vi "Directional Speed Sensor Page - Multi FPGA.vi"(8 "error in (no error)":errorcluster, 11 "Node Ptr":T1 format="%.0x") -> (0 "error out":errorcluster)   [LabVIEW 2015, in "Engine Simulation Toolkit System Explorer.lvlib"]
uses:
  <vilib>/NI Veristand/Custom Device API/Custom Device Item Ref.ctl
  Shared/Properties.vi
  Shared/Constants and GUIDs.vi
  <vilib>/NI Veristand/Custom Device Tools/Custom Device Utility Library/NI VeriStand - Search for All Items by GUID.vi
  <vilib>/NI Veristand/Custom Device API/Set Item Property (Dependent Node Pointer).vi
  <vilib>/NI Veristand/Custom Device API/Get Item Property (String).vi
  <vilib>/NI Veristand/Custom Device API/Get Item Property (Dependent Node Pointer).vi
  Engine Simulation Toolkit System Explorer.lvlib
  <vilib>/NI Veristand/Custom Device API/Custom Device API.lvlib
  Shared/Engine Simulation Toolkit Shared.lvlib
  <vilib>/NI Veristand/Custom Device Tools/Custom Device Utility Library/Custom Device Utility Library.lvlib
panel:
  in  "ToothSource":u16(ring) caption="Digital pattern to use for tooth centers"
  in  "Tr (uS)":dbl min=0.0 max=1638.4 step=0.025
  in  "Tf (uS)":dbl min=0.0 max=1638.4 step=0.025
  in  "Td (uS)":dbl min=0.0 max=1638.4 step=0.025
  out "Name in bitfile":string
  in  "Name":string
  in  "Header":cluster{"Section Name":string}={"Section Name"="Directional Speed Sensor Settings"}
  # "(Delay time)"
  # "(Forward pulse duration)"
  # "(Reverse pulse duration)"
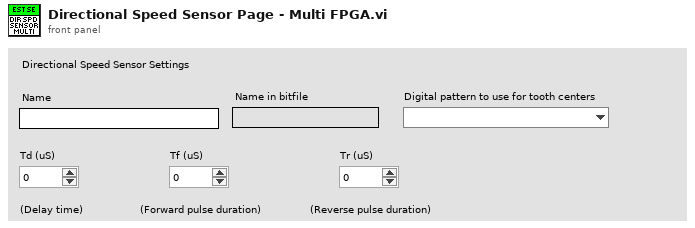
[diagram p1: front panel]
types:
  T1 = typedef "Custom Device API.lvlib/Custom Device Item Ref.ctl" = u64
  T2 = typedef "Engine Simulation Toolkit Shared.lvlib/Channel.ctl" = cluster{"Name":string, "Units":string, "Default":dbl, "Description":string, "Scalable":bool}
  T3 = typedef "Custom Device API.lvlib/Custom Device Item Info.ctl" = cluster{"Name":string, "Is Channel":bool, "GUID":string, "Is Waveform":bool}
  T4 = typedef "Custom Device API.lvlib/Custom Device Commands.ctl" = enum16{"Default", "Item renamed", "Shutdown", "Dynamic button pressed"}
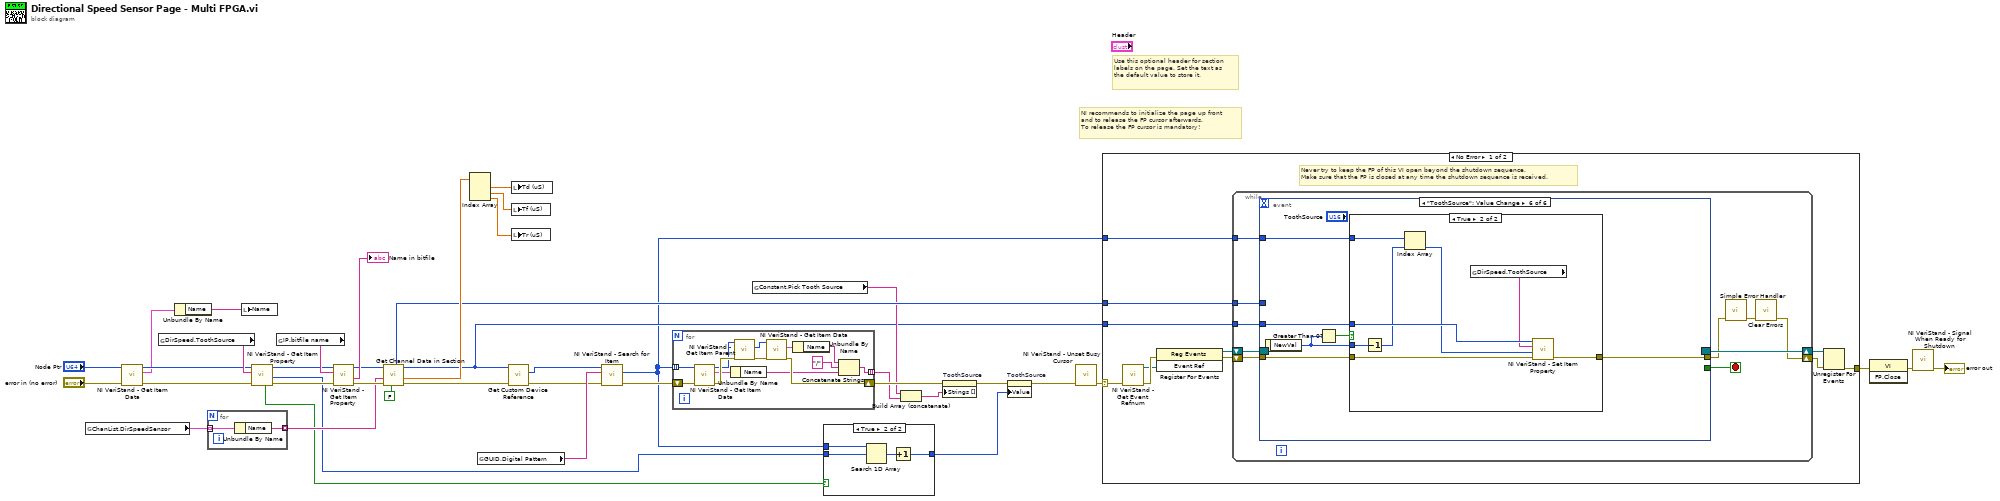
[diagram p0: block diagram]
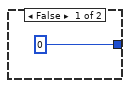
[diagram p2: hidden frame]
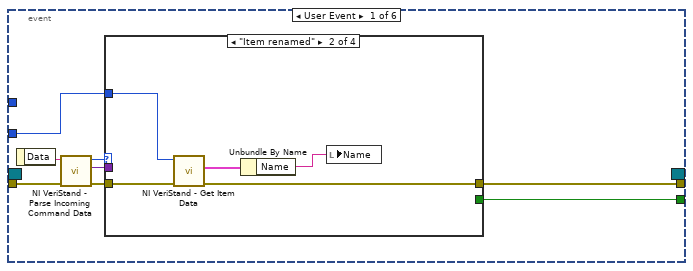
[diagram p3: hidden frame]
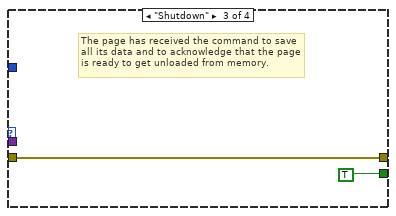
[diagram p5: hidden frame]
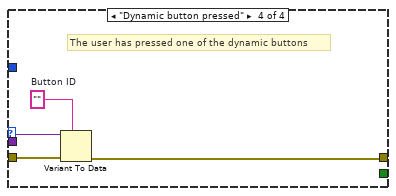
[diagram p6: hidden frame]
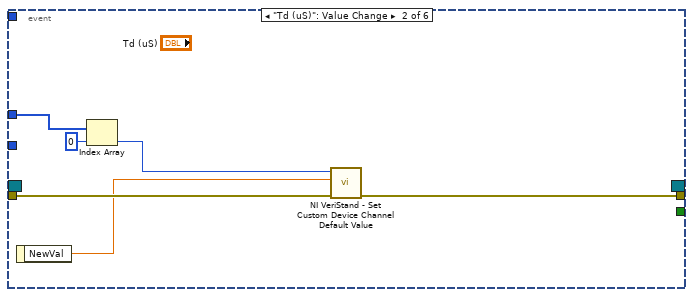
[diagram p7: hidden frame]
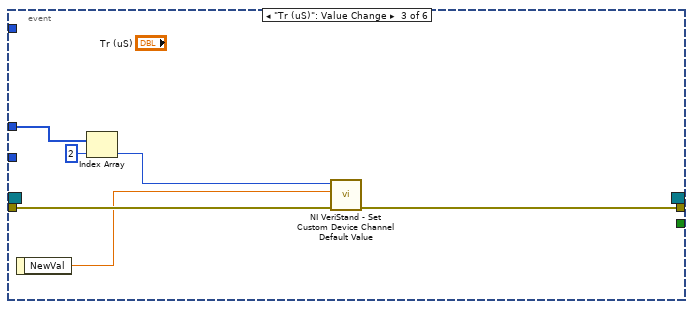
[diagram p8: hidden frame]
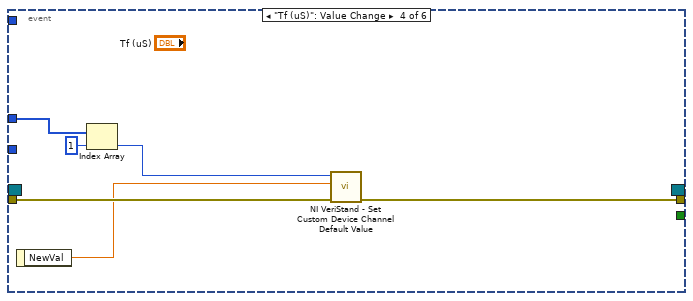
[diagram p9: hidden frame]
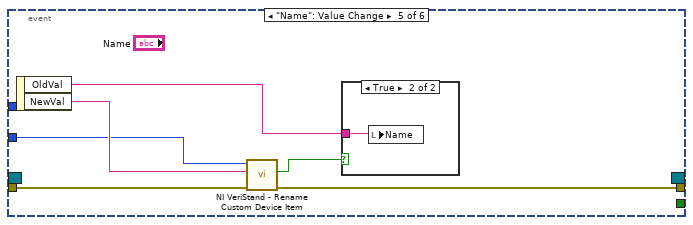
[diagram p10: hidden frame]
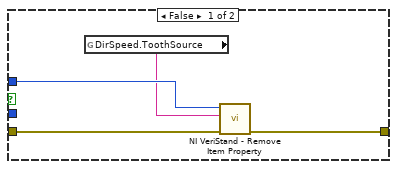
[diagram p12: hidden frame]
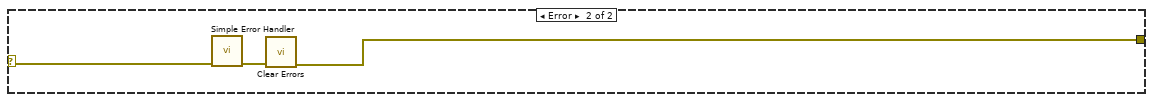
[diagram p13: hidden frame]
diagram:
  # "Use this optional header for section labels on the page. Set the text as the default value to store it."
  # "NI recommends to initialize the page up front\nand to release the FP cursor afterwards.\nTo release the FP cursor is mandatory!"
  n1 = global read "Constants and GUIDs.vi" "ChanList.DirSpeedSensor"() -> (w32:T2[])
  n2 = call <vilib>:"NI VeriStand - Get Item Data.vi"("error in (no error)"="error in (no error)", "Item Ref in"="Node Ptr") -> ("error out"=w10:errorcluster, "Item Info"=w7:T3, "Item Ref out"=w8:T1)  [unwired: 6 in, 1 out]
  n3 = global read "Properties.vi" "DirSpeed.ToothSource"() -> (w20:string)
  n4 = Unbundle By Name(w7) -> ("Name"=w6:string)
  n5 = for {
    tunnel: w32 -> [w43] mode=indexing
    tunnel: [w42] -> w31 mode=indexing
    n6 = Unbundle By Name(w43) -> ("Name"=w42:string)
  }
  n7 = local write "Name"(w6) -> ()
  n8 = call-poly <vilib>:"NI VeriStand - Get Item Property.vi"("error in (no error)"=w10, "Property Name"=w20, "Item Ref in"=w8) -> ("error out"=w22:errorcluster, "Dependent Node Ref"=w11:T1, "Item Ref out"=w21:T1, "Found"=w13:bool)  [unwired: 5 in]
  n9 = global read "Properties.vi" "IP.bitfile name"() -> (w36:string)
  n10 = call-poly <vilib>:"NI VeriStand - Get Item Property.vi"("error in (no error)"=w22, "Property Name"=w36, "Item Ref in"=w21) -> ("error out"=w34:errorcluster, "Value"=→"Name in bitfile":string, "Item Ref out"=w33:T1)  [unwired: 5 in, 1 out]
  n11 = call "Get Channel Data in Section.vi"("Get FIFO indexes (T)"=FALSE, "error in (no error)"=w34, "Channels"=w31, "Item Ref in"=w33) -> ("error out"=w4:errorcluster, "default values"=w29:dbl[], "Item Ref out"=w5:T1, "channel refs"=w25:T1[])  [unwired: 3 in, 1 out]
  n12 = Index Array(array=w29) -> (element #1=w28:dbl, element #2=w27:dbl, element #3=w26:dbl)  [unwired: 3 in]
  n13 = global read "Constants and GUIDs.vi" "GUID.Digital Pattern"() -> (w23:string)
  n14 = call "Get Custom Device Reference.vi"("error in (no error)"=w4, "Item Ref in"=w5) -> ("error out"=w3:errorcluster, "Custom Device Ref"=w2:T1)  [unwired: 7 in, 1 out]
  n15 = local write "Td (uS)"(w28) -> ()
  n16 = local write "Tf (uS)"(w27) -> ()
  n17 = local write "Tr (uS)"(w26) -> ()
  n18 = call-poly <vilib>:"NI VeriStand - Search for Item.vi"("error in"=w3, "Item GUID"=w23, "Section Ref in"=w2) -> ("error out"=w24:errorcluster, "Item Refs"=w1:T1[])  [unwired: 5 in, 2 out]
  n19 = for {
    shift-right: [w49] -> w19
    shift-left: w24 -> [w56]
    tunnel: w1 -> [w55] mode=indexing
    tunnel: [w47] -> w18 mode=indexing
    n20 = call <vilib>:"NI VeriStand - Get Item Data.vi"("error in (no error)"=w56, "Item Ref in"=w55) -> ("error out"=w54:errorcluster, "Item Info"=w52:T3, "Item Ref out"=w53:T1)  [unwired: 6 in, 1 out]
    n21 = Unbundle By Name(w52) -> ("Name"=w45:string)
    n22 = call <vilib>:"NI VeriStand - Get Item Parent.vi"("error in (no error)"=w54, "Item Ref in"=w53) -> ("error out"=w51:errorcluster, "Parent Ref"=w44:T1)  [unwired: 6 in, 2 out]
    n23 = call <vilib>:"NI VeriStand - Get Item Data.vi"("error in (no error)"=w51, "Item Ref in"=w44) -> ("error out"=w49:errorcluster, "Item Info"=w50:T3)  [unwired: 6 in, 2 out]
    n24 = Unbundle By Name(w50) -> ("Name"=w48:string)
    n25 = Concatenate Strings(w48, "/" ("string"), w45) -> (w47:string)
  }
  n26 = global read "Constants and GUIDs.vi" "Constant.Pick Tooth Source"() -> (w14:string)
  n27 = case shown="True" w13 {
    tunnel: w1 -> [_ w61]
    tunnel: [0 w59] -> w12
    tunnel: w11 -> [_ w58]
    frame False {
    }
    frame True {
      n28 = Search 1D Array(1D array=w61, element=w58) -> (index of element=w60:i32)  [unwired: 1 in]
      n29 = Increment(x=w60) -> (x+1=w59:i32)
    }
  }
  n30 = Build Array (concatenate)(w14, w18) -> (w15:string[])
  n31 = property on="ToothSource" class="Ring (strict)"(error in=w19, "Strings []"=w15) -> (error out=w17:errorcluster)  [unwired: 1 in, 1 out]
  n32 = property on="ToothSource" class="Ring (strict)"(error in=w17, "Value"=w12) -> (error out=w16:errorcluster)  [unwired: 1 in, 1 out]
  n33 = call <vilib>:"NI VeriStand - Unset Busy Cursor.vi"("error in (no error)"=w16) -> ("error out"=w38:errorcluster)  [unwired: 10 out]
  n34 = case shown="No Error" w38 {
    selector: w38 -> [w64 w148]
    tunnel: [w69 w146] -> w41
    tunnel: w5 -> [w65 _]
    tunnel: w25 -> [w63 _]
    tunnel: w1 -> [w62 _]
    frame No Error {
      # "Never try to keep the FP of this VI open beyond the shutdown sequence.\nMake sure that the FP is closed at any time the shutdown sequence is received."
      n35 = call <vilib>:"NI VeriStand - Get Event Refnum.vi"("error in (no error)"=w64) -> ("error out"=w72:errorcluster, "Event Ref"=w68:refnum<user-event>)  [unwired: 9 out]
      n36 = register-events(error in=w72, w68) -> (reference out=w66:refnum<event-registration>, error out=w67:errorcluster)  [unwired: 1 in]
      n37 = while {
        tunnel: w65 -> [w78]
        shift-right: [w75] -> w70
        shift-left: w67 -> [w81]
        shift-right: [w82] -> w71
        shift-left: w66 -> [w80]
        tunnel: w63 -> [w74]
        tunnel: w62 -> [w73]
        stop <- w79 stop-if-true
        n38 = event shown="[5] \"ToothSource\": Value Change" {
          selector: w80 -> [_ _ _ _ _ _]
          dyn-events: [_ _ _ _ _ _] -> w82
          timeout: _ -> [_ _ _ _ _ _]
          tunnel: w81 -> [w90 w108 w114 w120 w126 w133]
          tunnel: [w86 _ _ _ _ _] -> w79
          tunnel: [w85 w107 w113 w119 w125 w132] -> w77
          tunnel: w78 -> [w84 _ _ _ w123 w131]
          tunnel: w74 -> [_ w105 w111 w117 _ _]
          tunnel: w73 -> [_ _ _ _ _ w130]
          event User Event {
            n39 = event-data() -> ("Data"=w89:string)  [unwired: 1 out]
            n40 = call <vilib>:"NI VeriStand - Parse Incoming Command Data.vi"("error in (no error)"=w90, "Incoming data"=w89) -> ("error out"=w88:errorcluster, "Outgoing data"=w83:variant, "Action"=w87:T4)  [unwired: 7 out]
            n41 = case shown="\"Item renamed\"" w87 {
              tunnel: w88 -> [w91 w95 w97 w102]
              tunnel: [_ _ TRUE _] -> w86
              tunnel: [w91 w93 w97 w99] -> w85
              tunnel: w84 -> [_ w94 _ _]
              tunnel: w83 -> [_ _ _ w101]
              frame "Default", Default {
              }
              frame "Item renamed" {
                n42 = call <vilib>:"NI VeriStand - Get Item Data.vi"("error in (no error)"=w95, "Item Ref in"=w94) -> ("error out"=w93:errorcluster, "Item Info"=w96:T3)  [unwired: 8 out]
                n43 = Unbundle By Name(w96) -> ("Name"=w92:string)
                n44 = local write "Name"(w92) -> ()
              }
              frame "Shutdown" {
                # "The page has received the command to save all its data and to acknowledge that the page is ready to get unloaded from memory."
              }
              frame "Dynamic button pressed" {
                w100 = ""  # Button ID
                # "The user has pressed one of the dynamic buttons"
                n45 = Variant To Data(error in=w102, type=w100, Variant=w101) -> (error out=w99:errorcluster)  [unwired: 1 out]
              }
            }
          }
          event "Td (uS)": Value Change {
            n46 = event-data() -> ("NewVal"=w106:dbl)  [unwired: 1 out]
            n47 = Index Array(array=w105, index=0) -> (element=w104:T1)
            n48 = call <vilib>:"NI VeriStand - Set Custom Device Channel Default Value.vi"("error in (no error)"=w108, "Default Value"=w106, "Channel Ref in"=w104) -> ("error out"=w107:errorcluster)  [unwired: 7 in, 1 out]
          }
          event "Tr (uS)": Value Change {
            n49 = event-data() -> ("NewVal"=w112:dbl)  [unwired: 1 out]
            n50 = Index Array(array=w111, index=2) -> (element=w110:T1)
            n51 = call <vilib>:"NI VeriStand - Set Custom Device Channel Default Value.vi"("error in (no error)"=w114, "Default Value"=w112, "Channel Ref in"=w110) -> ("error out"=w113:errorcluster)  [unwired: 7 in, 1 out]
          }
          event "Tf (uS)": Value Change {
            n52 = event-data() -> ("NewVal"=w118:dbl)  [unwired: 1 out]
            n53 = Index Array(array=w117, index=1) -> (element=w116:T1)
            n54 = call <vilib>:"NI VeriStand - Set Custom Device Channel Default Value.vi"("error in (no error)"=w120, "Default Value"=w118, "Channel Ref in"=w116) -> ("error out"=w119:errorcluster)  [unwired: 7 in, 1 out]
          }
          event "Name": Value Change {
            n55 = event-data() -> ("OldVal"=w121:string, "NewVal"=w124:string)  [unwired: 1 out]
            n56 = call <vilib>:"NI VeriStand - Rename Custom Device Item.vi"("error in (no error)"=w126, "New Name"=w124, "Item Ref in"=w123) -> ("error out"=w125:errorcluster, "Request invalid?"=w122:bool)  [unwired: 1 in, 6 out]
            n57 = case shown="True" w122 {
              tunnel: w121 -> [_ w127]
              frame False {
              }
              frame True {
                n58 = local write "Name"(w127) -> ()
              }
            }
          }
          event "ToothSource": Value Change {
            n59 = event-data() -> ("NewVal"=w128:u16)  [unwired: 1 out]
            n60 = Greater Than 0?(x=w128) -> (x > 0?=w129:bool)
            n61 = case shown="True" w129 {
              tunnel: w133 -> [w137 w145]
              tunnel: [w136 w144] -> w132
              tunnel: w131 -> [w135 w143]
              tunnel: w128 -> [_ w142]
              tunnel: w130 -> [_ w141]
              frame False {
                n62 = global read "Properties.vi" "DirSpeed.ToothSource"() -> (w134:string)
                n63 = call <vilib>:"NI VeriStand - Remove Item Property.vi"("error in (no error)"=w137, "Property Name"=w134, "Item Ref in"=w135) -> ("error out"=w136:errorcluster)  [unwired: 6 in, 2 out]
              }
              frame True {
                n64 = Decrement(x=w142) -> (x-1=w140:u16)
                n65 = Index Array(array=w141, index=w140) -> (element=w139:T1)
                n66 = global read "Properties.vi" "DirSpeed.ToothSource"() -> (w138:string)
                n67 = call-poly <vilib>:"NI VeriStand - Set Item Property.vi"("error in (no error)"=w145, "Dependent Node Ref"=w139, "Property Name"=w138, "Item Ref in"=w143) -> ("error out"=w144:errorcluster)  [unwired: 5 in, 2 out]
              }
            }
          }
        }
        n68 = call <vilib>:"Simple Error Handler.vi"("error in (no error)"=w77) -> ("error out"=w76:errorcluster)  [unwired: 1 in, 7 out]
        n69 = call <vilib>:"Clear Errors.vi"("error in (no error)"=w76) -> ("error out"=w75:errorcluster)  [unwired: 1 in, 5 out]
      }
      n70 = Unregister For Events(event registration refnum=w71, error in=w70) -> (error out=w69:errorcluster)
    }
    frame Error {
      n71 = call <vilib>:"Simple Error Handler.vi"("error in (no error)"=w148) -> ("error out"=w147:errorcluster)  [unwired: 1 in, 7 out]
      n72 = call <vilib>:"Clear Errors.vi"("error in (no error)"=w147) -> ("error out"=w146:errorcluster)  [unwired: 1 in, 5 out]
    }
  }
  n73 = invoke class="VI" method="FP.Close"(error in=w41) -> (error out=w40:errorcluster)  [unwired: 2 in, 2 out]
  n74 = call <vilib>:"NI VeriStand - Signal When Ready for Shutdown.vi"("error in (no error)"=w40) -> ("error out"=→"error out":errorcluster)  [unwired: 10 out]
